vi "TEST - Get TDEnum from Data.vi"(8 "error in (no error)":errorcluster) -> (0 "error out":errorcluster, 2 "pass":bool)   [LabVIEW 2013]
uses:
  source/library/Type Descriptor Enumeration.ctl
panel:
  out "Failures":T2(array[cluster]) {"result"."Type Descriptor Enumeration" format="%.0x"; "exected result"."Type Descriptor Enumeration" format="%.0x"}
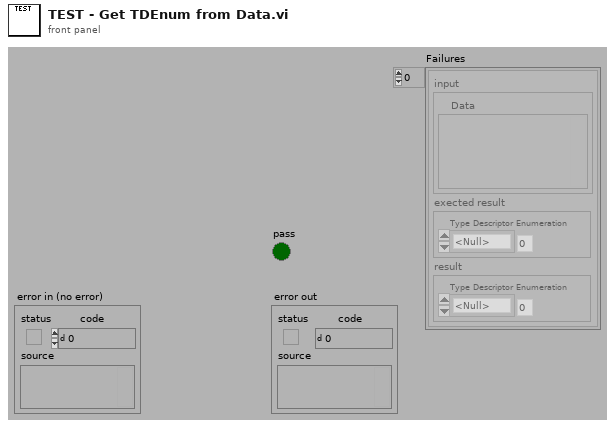
[diagram p1: front panel]
types:
  T1 = typedef "Type Descriptor Enumeration.ctl" = enum8{"<Null>", "I8", "I16", "I32", "I64", "U8", "U16", "U32", "U64", "SGL", "DBL", "EXT", "CSG", "CDB", "CXT", "0x0F", "0x10", "0x11", "0x12", "0x13", "0x14", "Enum U8", "Enum U16", "Enum U32", "Enum U64", "SGL PQ", "DBL PQ", "EXT PQ", "CSG PQ", "CDB PQ", "CXT PQ", "0x1F", "0x20", "Boolean", "0x22", "0x23", "0x24", "0x25", "0x26", "0x27", "0x28", "0x29", "0x2A", "0x2B", "0x2C", "0x2D", "0x2E", "0x2F", "String", "0x31", "Path", "Pict", "0x34", "0x35", "0x36", "DAQ", "0x38", "0x39", "0x3A", "0x3B", "0x3C", "0x3D", "0x3E", "0x3F", "Array", "0x41", "0x42", "0x43", "0x44", "0x45", "0x46", "0x47", "0x48", "0x49", "0x4A", "0x4B", "0x4C", "0x4D", "0x4E", "0x4F", "Cluster", "0x51", "0x52", "Variant", "Waveform", "0x55", "0x56", "0x57", "0x58", "0x59", "0x5A", "0x5B", "0x5C", "0x5D", "0x5E", "Fixed Point", "0x60", "0x61", "0x62", "0x63", "0x64", "0x65", "0x66", "0x67", "0x68", "0x69", "0x6A", "0x6B", "0x6C", "0x6D", "0x6E", "0x6F", "Refnum", "0x71", "0x72", "Set Collection", "Map Collection"}
  T2 = cluster{"input":cluster{"Data":variant}, "exected result":cluster{"Type Descriptor Enumeration":T1}, "result":cluster{"Type Descriptor Enumeration":T1}}[]
  T3 = cluster{"input":cluster{"Data":variant}, "exected result":cluster{"Type Descriptor Enumeration":T1}, "result":cluster{"Type Descriptor Enumeration":T1}}
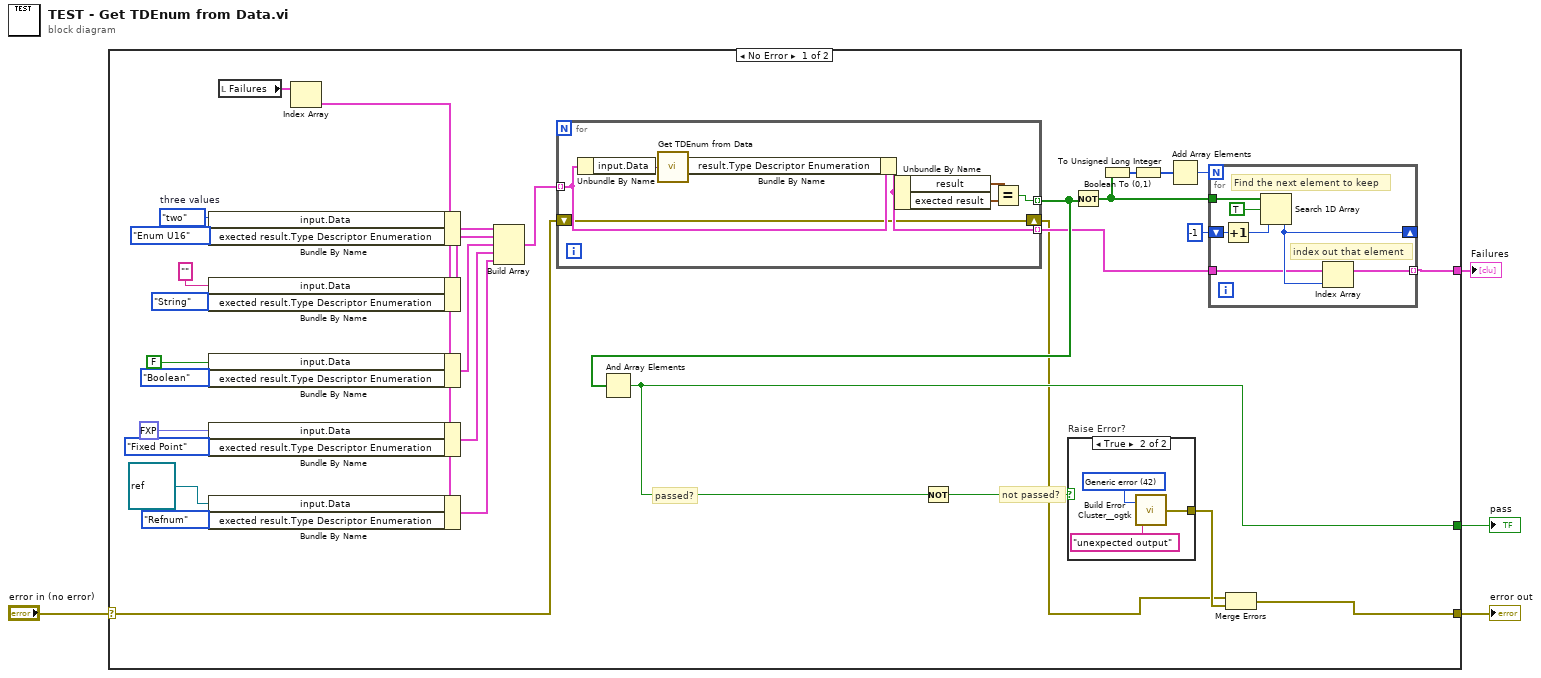
[diagram p0: block diagram]
diagram:
  n1 = case shown="No Error" "error in (no error)" {
    selector: "error in (no error)" -> [w22 w55]
    tunnel: [w33 _] -> w4
    tunnel: [w36 w55] -> w2
    tunnel: [w25 _] -> w1
    frame No Error {
      w19 = enum16{"one", "two", "three"}."two"  # three values
      # "not passed?"
      # "passed?"
      n2 = local read "Failures"() -> (w20:T2)
      n3 = Index Array(array=w20) -> (element=w5:T3)  [unwired: 1 in]
      n4 = Bundle By Name(cluster=w5, "input.Data"=w19, "exected result.Type Descriptor Enumeration"=Type_Descriptor_Enumeration."Enum U16") -> (w24:T3)
      n5 = Bundle By Name(cluster=w5, "input.Data"="", "exected result.Type Descriptor Enumeration"=Type_Descriptor_Enumeration."String") -> (w15:T3)
      n6 = Bundle By Name(cluster=w5, "input.Data"=FALSE, "exected result.Type Descriptor Enumeration"=Type_Descriptor_Enumeration."Boolean") -> (w14:T3)
      n7 = Bundle By Name(cluster=w5, "input.Data"=fxp<+,1,1> 0.0, "exected result.Type Descriptor Enumeration"=Type_Descriptor_Enumeration."Fixed Point") -> (w9:T3)
      n8 = Bundle By Name(cluster=w5, "input.Data"=refnum<class> refnum ("LabVIEW Object"), "exected result.Type Descriptor Enumeration"=Type_Descriptor_Enumeration."Refnum") -> (w6:T3)
      n9 = Build Array(w24, w15, w14, w9, w6) -> (w23:T2)
      n10 = for {
        tunnel: w23 -> [w50] mode=indexing
        tunnel: [w51] -> w27 mode=indexing
        tunnel: [w49] -> w26 mode=indexing
        shift-right: [w44] -> w21
        shift-left: w22 -> [w44]
        n11 = Unbundle By Name(w50) -> ("input.Data"=w46:variant)
        n12 = call "Get TDEnum from Data.vi"("Data"=w46) -> ("Type Descriptor Enumeration"=w45:T1)  [unwired: 4 in]
        n13 = Bundle By Name(cluster=w50, "result.Type Descriptor Enumeration"=w45) -> (w49:T3)
        n14 = Unbundle By Name(w49) -> ("result"=w48:cluster{"Type Descriptor Enumeration":T1}, "exected result"=w47:cluster{"Type Descriptor Enumeration":T1})
        n15 = Equal?(x=w48, y=w47) -> (x = y?=w51:bool)
      }
      n16 = And Array Elements(Boolean array=w27) -> (logical AND=w33:bool)
      n17 = Not(x=w33) -> (.not. x?=w34:bool)
      n18 = case "Raise Error?" shown="True" w34 {
        tunnel: [_ w52] -> w35
        frame False {
        }
        frame True {
          w53 = 42 items=["No error", "Argument error", "Memory is full", "Out of zone", "End of file", "File already open", "Generic file I/O error", "File not found", "File permission error", "Disk is full", "Duplicate path", "Too many files open", "System feature not enabled", "Resource file not found", "Cannot add resource", "Resource not found", "Image not found", "Image memory error", "Pen does not exist", "Config type invalid", "Config token not found", "Config parse error", "Config memory error", "Bad external code format", "Bad external code offset", "External code not present", "Null window", "Destroy window error", "Null menu", "Print aborted", "Bad print record", "Print driver error", "Windows error during printing", "Memory error during printing", "Print dialog error", "Generic print error", "Invalid device refnum", "Device not found", "Device parameter error", "Device unit error", "Cannot open device", "Device call aborted", "Generic error", "Cancelled by user", "Object ID too low", "Object ID too high", "Object not in heap", "Unknown heap", "Unknown object (invalid DefProc)", "Unknown object (DefProc not in table)", "Message out of range", "Invalid (null) method", "Unknown message", "Manager call not supported", "Bad address", "Network operation in progress", "Network operation timed out", "Connection is busy", "Network attribute not supported", "Network error", "Address in use", "System out of memory", "Connection aborted", "Connection refused", "Not connected", "Already connected", "Connection closed", "Initialization error (interapplication manager)", "Bad occurrence", "Wait on unbound occurrence handler", "Occurrence queue overflow", "Datalog type conflict", "Unused", "Unrecognized type (interapplication manager)", "Memory corrupt", "Failed to make temporary DLL", "Old CIN version", "Drag socket not found", "Failed to load drop-object", "Failed to register OLE object", "Failed to release OLE object", "Format specifier type mismatch", "Unknown format specifier", "Too few format specifiers", "Too many format specifiers", "Scan failed", "Newer CIN version", "Error converting to variant", "Runtime menu error", "Password tampered", "Variant attribute not found", "Incompatible variant data type", "Event data is not available", "Event Store is not present", "Occurrence is not found", "Event Queue is not created", "Event info is not available", "Refnum passed is NULL", "Error retrieving Class GUID", "Error retrieving CoClass GUID", "Error retrieving TypeLib GUID.", "Bad built application magic bytes.", "Specific driver is different from the specific driver associated with the Logical Name.", "There is no session opened to the class driver.", "Max Error", "MAX - Error with config objects", "MAX - Error loading configuration", "MAX - Group not supported"]
          n19 = call <userlib>:"Build Error Cluster__ogtk.vi"("String to Prepend to source (\"\")"="unexpected output" ("String to Prepend to source (\"\")"), "code"=w53) -> ("error out"=w52:errorcluster)
        }
      }
      n20 = Not(x=w27) -> (.not. x?=w29:bool[])
      n21 = Boolean To (0,1)(Boolean=w29) -> (0, 1=w30:i16[])
      n22 = To Unsigned Long Integer(number=w30) -> (unsigned 32bit integer=w28:u32[])
      n23 = Add Array Elements(numeric array=w28) -> (sum=w31:u32)
      n24 = for {
        N: w31 -> [_]
        tunnel: w26 -> [w39]
        tunnel: w29 -> [w43]
        shift-right: [w40] -> _
        shift-left: -1 ("start index (0)") -> [w41]
        tunnel: [w38] -> w25 mode=indexing
        # "index out that element"
        # "Find the next element to keep"
        n25 = Increment(x=w41) -> (x+1=w37:i32)
        n26 = Search 1D Array(1D array=w43, element=TRUE, start index (0)=w37) -> (index of element=w40:i32)
        n27 = Index Array(array=w39, index=w40) -> (element=w38:T3)
      }
      n28 = Merge Errors(w21, w35) -> (w36:errorcluster)
    }
    frame Error {
    }
  }
  "pass" <- w4
  "error out" <- w2
  "Failures" <- w1
